vi "Clear Tree.vi"(8 "error in (no error)":errorcluster, 11 "Tag Tree In":refnum<class "Tag Tree.lvclass">) -> (0 "error out":errorcluster, 3 "Tag Tree Out":refnum<class "Tag Tree.lvclass">)   [LabVIEW 2020, in "Tag Tree.lvclass"]
uses:
  Tag Tree.lvclass
  Tag Tree.lvclass/Tag Tree.ctl
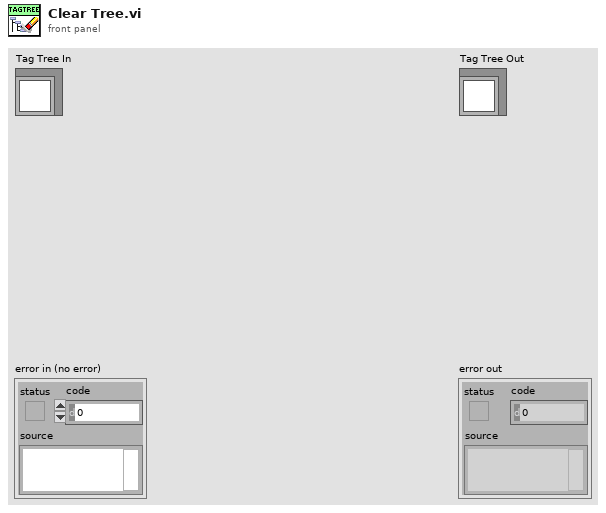
[diagram p1: front panel]
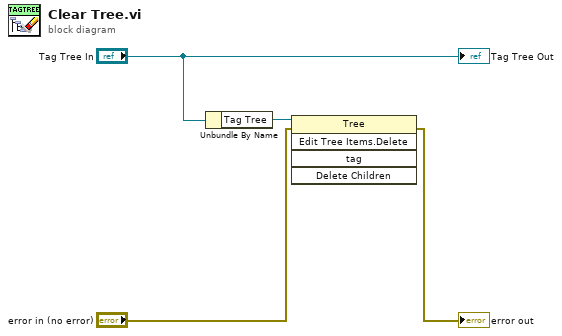
[diagram p0: block diagram]
diagram:
  n1 = Unbundle By Name("Tag Tree In") -> ("Tag Tree"=w3:refnum<vi>)
  n2 = invoke class="Tree" method="Edit Tree Items.Delete"(reference=w3, error in="error in (no error)") -> (error out=→"error out":errorcluster)  [unwired: 3 in, 4 out]
  "Tag Tree Out" <- "Tag Tree In"
